vi "SPARK Get Status 7.vi"(8 "error in (no error)":errorcluster, 11 "MotorControlDeviceRef in":T2={"DeviceStatus"={"status"=FALSE, "code"=0, "source"=""}, "Type"=enum."PWM", "PWM"={"PWM Channel"=enum."Invalid", "DeadBand"={"Name"="", "maxPositivePwm"=0, "minPositivePwm"=0, "centerPwm"=0, "maxNegativePwm"=0, "minNegativePwm"=0, "angularRange"=0}}, "CAN"={"Device Number"=0, "SetOutput VI Ref"=variant, "GetOutput VI Ref"=variant, "Enable VI Ref"=variant, "Disable VI Ref"=variant, "Data"=variant}, "Invert"=FALSE, "DIO PWM"={"PWM \"Enable\" Channel"=enum."Invalid", "DIOChannel"=enum."Invalid", "PWM Rate"=0.0}}) -> (0 "error out":errorcluster, 2 "Status 7 Frame":T1, 3 "MotorControlDeviceRef out":T2={"DeviceStatus"={"status"=FALSE, "code"=0, "source"=""}, "Type"=enum."PWM", "PWM"={"PWM Channel"=enum."Invalid", "DeadBand"={"Name"="", "maxPositivePwm"=0, "minPositivePwm"=0, "centerPwm"=0, "maxNegativePwm"=0, "minNegativePwm"=0, "angularRange"=0}}, "CAN"={"Device Number"=0, "SetOutput VI Ref"=variant, "GetOutput VI Ref"=variant, "Enable VI Ref"=variant, "Disable VI Ref"=variant, "Data"=variant}, "Invert"=FALSE, "DIO PWM"={"PWM \"Enable\" Channel"=enum."Invalid", "DIOChannel"=enum."Invalid", "PWM Rate"=0.0}})   [LabVIEW 2023]
uses:
  <vilib>/Rock Robotics/WPI/MotorControl/WPI_MotorControlDeviceRef.ctl
  <vilib>/Rock Robotics/WPI/MotorControl/WPI_MotorControlType.ctl
  <vilib>/Rock Robotics/SystemInterfaces/DIO/FPGA_DIOPWMChannel.ctl
  <vilib>/Rock Robotics/WPI/PWM/WPI_PWMDeadband.ctl
  <vilib>/Rock Robotics/SystemInterfaces/DIO/FPGA_DIOChannel.ctl
  Typedef/SPARK Status 7 Frame.ctl
  Typedef/Spark MAX Variant Data.ctl
  Typedef/SPARK Model.ctl
  Typedef/SPARK CAN Arb ID.ctl
  Typedef/SPARK Periodic Status.ctl
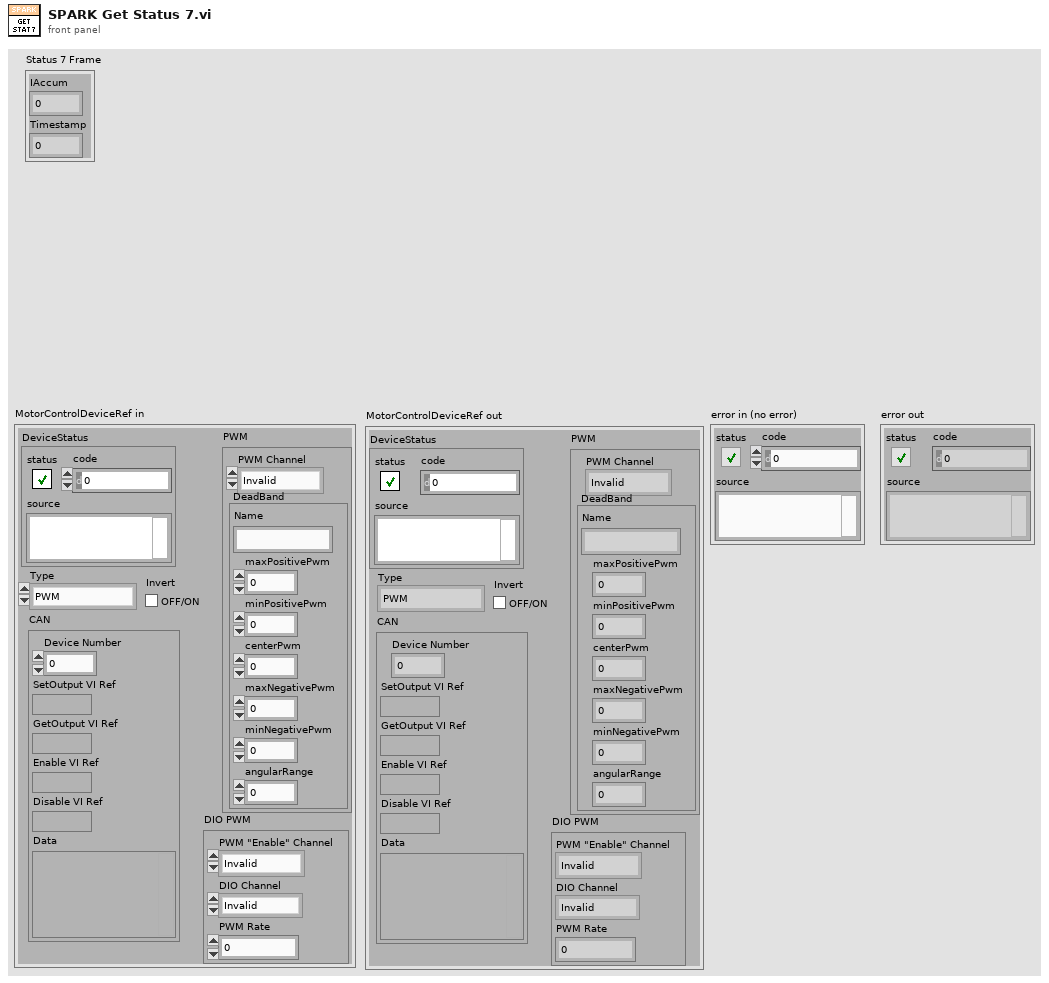
[diagram p1: front panel]
types:
  T1 = typedef "SPARK Status 7 Frame.ctl" = cluster{"IAccum":dbl, "Timestamp":u32}
  T2 = typedef "WPI_MotorControlDeviceRef.ctl" = cluster{"DeviceStatus":errorcluster, "Type":T3, "PWM":cluster{"PWM Channel":T4, "DeadBand":T5}, "CAN":cluster{"Device Number":u8, "SetOutput VI Ref":variant, "GetOutput VI Ref":variant, "Enable VI Ref":variant, "Disable VI Ref":variant, "Data":variant}, "Invert":bool, "DIO PWM":cluster{"PWM \"Enable\" Channel":T4, "DIOChannel":T6, "PWM Rate":dbl}}
  T3 = typedef "WPI_MotorControlType.ctl" = enum16{"PWM", "CAN", "DIO PWM"}
  T4 = typedef "FPGA_DIOPWMChannel.ctl" = enum8{"PWM 0", "PWM 1", "PWM 2", "PWM 3", "PWM 4", "PWM 5", "PWM 6", "PWM 7", "PWM 8", "PWM 9", "PWM MXP 0", "PWM MXP 1", "PWM MXP 2", "PWM MXP 3", "PWM MXP 4", "PWM MXP 5", "PWM MXP 6", "PWM MXP 7", "PWM MXP 8", "PWM MXP 9", "Invalid"}
  T5 = typedef "WPI_PWMDeadband.ctl" = cluster{"Name":string, "maxPositivePwm":i32, "minPositivePwm":i32, "centerPwm":i32, "maxNegativePwm":i32, "minNegativePwm":i32, "angularRange":u16}
  T6 = typedef "FPGA_DIOChannel.ctl" = enum8{"DIO 0", "DIO 1", "DIO 2", "DIO 3", "DIO 4", "DIO 5", "DIO 6", "DIO 7", "DIO 8", "DIO 9", "DIO MXP 0", "DIO MXP 1", "DIO MXP 2", "DIO MXP 3", "DIO MXP 4", "DIO MXP 5", "DIO MXP 6", "DIO MXP 7", "DIO MXP 8", "DIO MXP 9", "DIO MXP 10", "DIO MXP 11", "DIO MXP 12", "DIO MXP 13", "DIO MXP 14", "DIO MXP 15", "SPI Port CS1", "SPI Port CS2", "SPI Port CS3", "SPI Port MISO", "SPI Port MOSI", "Invalid"}
  T7 = typedef "SPARK Periodic Status.ctl" = enum16{"Periodic Status 0", "Periodic Status 1", "Periodic Status 2", "Periodic Status 3", "Periodic Status 4", "Periodic Status 5", "Periodic Status 6", "Periodic Status 7"}
  T8 = typedef "SPARK CAN Arb ID.ctl" = u32
  T9 = typedef "Spark MAX Variant Data.ctl" = cluster{"Ext ID":u32, "CAN Timeout":u32, "Inverted No WPILib":bool, "Has Configured Limit Sw":bool, "Has Configured Alt Encoder":bool, "SPARK Model":T10, "CAN Max Retries":u32, "CAN Timeout (ms)":u32, "Status 0 Period (ms)":u32, "Status 1 Period (ms)":u32, "Status 2 Period (ms)":u32, "Status 3 Period (ms)":u32, "Status 4 Period (ms)":u32, "Status 5 Period (ms)":u32, "Status 6 Period (ms)":u32, "Status 7 Period (ms)":u32, "Status Frame Timeout (ms)":u32}
  T10 = typedef "SPARK Model.ctl" = enum16{"SPARK MAX", "SPARK Flex", "Unknown"}
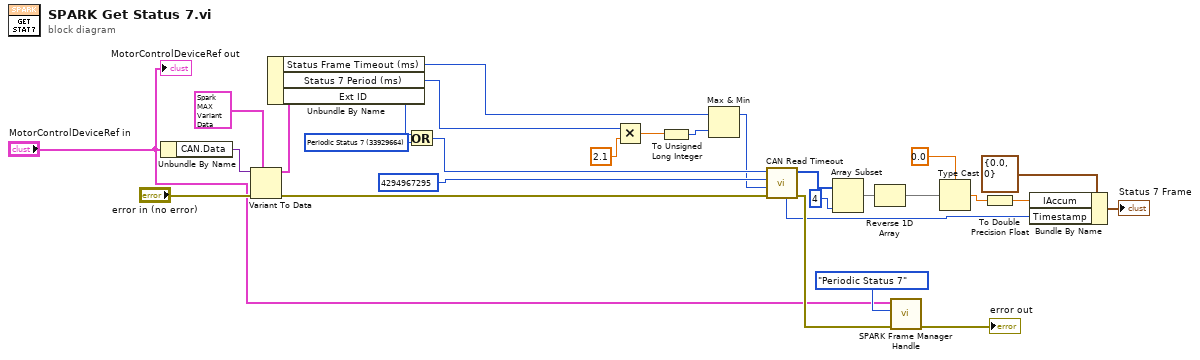
[diagram p0: block diagram]
diagram:
  w24 = T8 33929664 items=["Broadcast Disable"=0, "Broadcast System Halt"=64, "Broadcast System Reset"=128, "Broadcast Device Assign"=192, "Broadcast Heartbeat"=320, "Broadcast Firmware Version"=512, "Broadcast Enumerate"=576, "Broadcast System Resume"=640, "Velocity Setpoint"=33882112, "Duty Cycle Setpoint"=33882240, "Smart Velocity Setpoint"=33882304, "Position Setpoint"=33882368, "Voltage Setpoint"=33882432, "Current Setpoint"=33882496, "Smart Motion Setpoint"=33882560, "MAXMotion Position Setpoint"=33882624, "MAXMotion Velocity Setpoint"=33882688, "Periodic Status 0"=33929216, "Periodic Status 1"=33929280, "Periodic Status 2"=33929344, "Periodic Status 3"=33929408, "Periodic Status 4"=33929472, "Periodic Status 5"=33929536, "Periodic Status 6"=33929600, "Periodic Status 7"=33929664, "Set Statuses Enabled"=33883136, "Set Statuses Enabled Response"=33883200, "DRV Status"=33888896, "Clear Faults"=33889152, "Parameter Write"=33896448, "Parameter Write Response"=33896512, "Parameter Double Read Start (RTR)"=33897472, "Config Burn Flash"=33889408, "Set Follower Mode"=33889472, "Config Factory Defaults"=33889536, "Config Factory Reset"=33889600, "Nack"=33890304, "Ack"=33890368, "Broadcast (not a command)"=33891328, "Heartbeat"=33891456, "Sync"=33891520, "IDQuery"=33891584, "IDAssign"=33891648, "Firmware Version"=33891840, "REV Enumerate"=33891904, "Legacy/USB Heartbeat"=33891968, "roboRIO Lock"=33892032, "SWDL Data"=33892096, "SWDL Checksum"=33892160, "SWDL Retransmit"=33892224, "Telemetry Update Mechanical Position Enoder Port"=33892352, "Telemetry Update I Accum"=33892480, "Telemtry Update Mechanical Position Alt Encoder"=33892608, "Telemetry Update Mechanical Position Analog"=33892544, "Non-roboRIO Broadcast (not a command)"=33893376, "non-RIO Lock"=33893440, "non-RIO Heartbeat"=33893504] ("Parameter ID")
  n1 = Unbundle By Name("MotorControlDeviceRef in") -> ("CAN.Data"=w29:variant)
  n2 = Variant To Data(error in="error in (no error)", type=T9 {"Ext ID"=0, "CAN Timeout"=0, "Inverted No WPILib"=FALSE, "Has Configured Limit Sw"=FALSE, "Has Configured Alt Encoder"=FALSE, "SPARK Model"=enum."Unknown", "CAN Max Retries"=5, "CAN Timeout (ms)"=20, "Status 0 Period (ms)"=10, "Status 1 Period (ms)"=250, "Status 2 Period (ms)"=20, "Status 3 Period (ms)"=20, "Status 4 Period (ms)"=20, "Status 5 Period (ms)"=20, "Status 6 Period (ms)"=20, "Status 7 Period (ms)"=20, "Status Frame Timeout (ms)"=500} ("SPARK MAX Device Ref"), Variant=w29) -> (data=w26:T9, error out=w21:errorcluster)
  n3 = Unbundle By Name(w26) -> ("Status Frame Timeout (ms)"=w1:u32, "Status 7 Period (ms)"=w2:u32, "Ext ID"=w25:u32)
  n4 = Or(x=w25, y=w24) -> (x .or. y?=w23:T8)
  n5 = Multiply(x=w2, y=2.1) -> (x*y=w5:dbl)
  n6 = To Unsigned Long Integer(number=w5) -> (unsigned 32bit integer=w4:u32)
  n7 = Max & Min(x=w1, y=w4) -> (max(x,y)=w3:u32)  [unwired: 1 out]
  n8 = call "CAN Read Timeout.vi"("error in (no error)"=w21, "Timeout (ms)"=w3, "Message ID Mask"=u32 4294967295, "Message ID"=w23) -> ("error out"=w11:errorcluster, "data"=w14:u8[], "timestamp"=w8:u32)  [unwired: 5 in]
  n9 = Array Subset(array=w14, length=4) -> (w20:u8[])  [unwired: 1 in]
  n10 = Reverse 1D Array(array=w20) -> (reversed array=w19:u8[])
  n11 = call "SPARK Frame Manager Handle.vi"("error in (no error)"=w11, "Periodic Status"=SPARK_Periodic_Status."Periodic Status 7", "MotorControlDeviceRef"="MotorControlDeviceRef in") -> ("error out"=→"error out":errorcluster)  [unwired: 8 in]
  n12 = Type Cast(type=sgl 0.0, x=w19) -> (*(type *) &x=w17:sgl)
  n13 = To Double Precision Float(number=w17) -> (double precision float=w16:dbl)
  n14 = Bundle By Name(cluster=T1 {"IAccum"=0.0, "Timestamp"=0} ("Status 7 Frame"), "IAccum"=w16, "Timestamp"=w8) -> (→"Status 7 Frame":T1)
  "MotorControlDeviceRef out" <- "MotorControlDeviceRef in"
